vi "FPGA Output Read.vi"(8 "error in (no error)":errorcluster, 10 "Output Register Info":T2, 11 "FPGA Session In":refnum<class "FPGA Interface Base.lvclass">) -> (0 "error out":errorcluster, 2 "Data":dbl, 3 "FPGA Session Out":refnum<class "FPGA Interface Base.lvclass">)   [LabVIEW 2010, in "Sensor Simulation Custom Device.lvlib"]
uses:
  Sensor Simulation Custom Device.lvlib
  <userlib>/_FPGA Interface Advanced Tools/FPGA Interface Base/FPGA Interface Base.lvclass
  TypeDefs/OutputChannelTypes.ctl
  <userlib>/_FPGA Interface Advanced Tools/FPGA Interface Base/FPGA Read By Name - U64.vi
  <userlib>/_FPGA Interface Advanced Tools/FPGA Interface Base/FPGA Read By Name - U32.vi
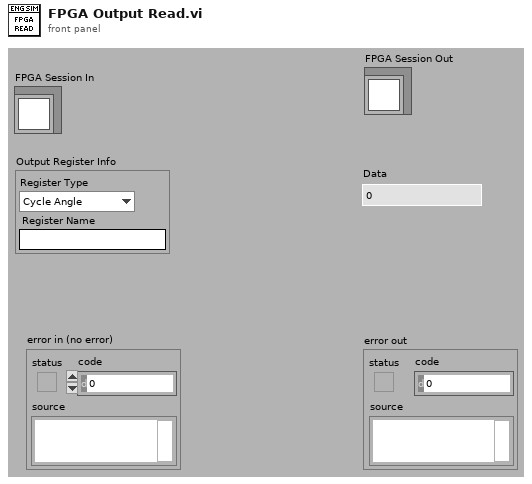
[diagram p1: front panel]
types:
  T1 = typedef "Sensor Simulation Custom Device.lvlib/OutputChannelTypes.ctl" = enum16{"Cycle Angle", "Crank Angle", "Time Duration", "Angle Duration", "Start Angle", "End Angle"}
  T2 = cluster{"Register Type":T1, "Register Name":string}
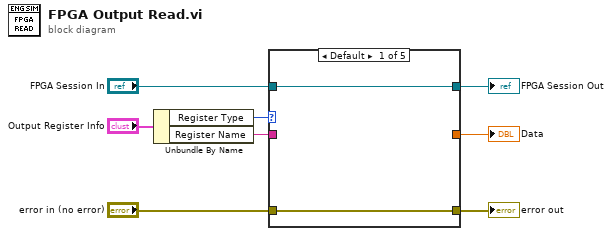
[diagram p0: block diagram]
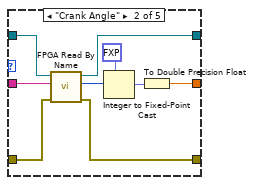
[diagram p2: hidden frame]
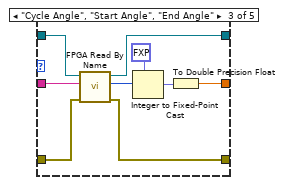
[diagram p3: hidden frame]
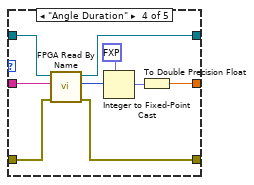
[diagram p4: hidden frame]
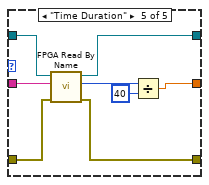
[diagram p5: hidden frame]
diagram:
  n1 = Unbundle By Name("Output Register Info") -> ("Register Type"=w7:T1, "Register Name"=w6:string)
  n2 = case shown="Default" w7 {
    tunnel: w6 -> [_ w18 w27 w36 w44]
    tunnel: "FPGA Session In" -> [w10 w19 w28 w37 w45]
    tunnel: [w10 w16 w25 w34 w42] -> w4
    tunnel: "error in (no error)" -> [w9 w17 w26 w35 w43]
    tunnel: [w9 w15 w24 w33 w41] -> w2
    tunnel: [_ w11 w20 w29 w38] -> w1
    frame Default {
    }
    frame "Crank Angle" {
      n3 = call-poly <userlib>:"FPGA Read By Name.vi"("error in (no error)"=w17, "Indicator"=w18, "FPGA Session In"=w19) -> ("error out"=w15:errorcluster, "Value"=w14:u64, "FPGA Session Out"=w16:refnum<class "FPGA Interface Base.lvclass">)  [unwired: 6 in]
      n4 = Integer to Fixed-Point Cast(fixed-point type=fxp<+,60,9> 0.0, integer=w14) -> (fixed-point=w12:fxp<+,60,9>)
      n5 = To Double Precision Float(number=w12) -> (double precision float=w11:dbl)
    }
    frame "Cycle Angle", "Start Angle", "End Angle" {
      n6 = call-poly <userlib>:"FPGA Read By Name.vi"("error in (no error)"=w26, "Indicator"=w27, "FPGA Session In"=w28) -> ("error out"=w24:errorcluster, "Value"=w23:u64, "FPGA Session Out"=w25:refnum<class "FPGA Interface Base.lvclass">)  [unwired: 6 in]
      n7 = Integer to Fixed-Point Cast(fixed-point type=fxp<+,61,10> 0.0, integer=w23) -> (fixed-point=w21:fxp<+,61,10>)
      n8 = To Double Precision Float(number=w21) -> (double precision float=w20:dbl)
    }
    frame "Angle Duration" {
      n9 = call-poly <userlib>:"FPGA Read By Name.vi"("error in (no error)"=w35, "Indicator"=w36, "FPGA Session In"=w37) -> ("error out"=w33:errorcluster, "Value"=w32:u64, "FPGA Session Out"=w34:refnum<class "FPGA Interface Base.lvclass">)  [unwired: 6 in]
      n10 = Integer to Fixed-Point Cast(fixed-point type=fxp<+/-,62,11> 0.0, integer=w32) -> (fixed-point=w30:fxp<+/-,62,11>)
      n11 = To Double Precision Float(number=w30) -> (double precision float=w29:dbl)
    }
    frame "Time Duration" {
      n12 = call-poly <userlib>:"FPGA Read By Name.vi"("error in (no error)"=w43, "Indicator"=w44, "FPGA Session In"=w45) -> ("error out"=w41:errorcluster, "Value"=w40:u32, "FPGA Session Out"=w42:refnum<class "FPGA Interface Base.lvclass">)  [unwired: 6 in]
      n13 = Divide(x=w40, y=u32 40) -> (x/y=w38:dbl)
    }
  }
  "FPGA Session Out" <- w4
  "Data" <- w1
  "error out" <- w2
